vi "SlaveAccelerometerSample6.vi"   [LabVIEW 2016]
uses:
  <vilib>/rvi/Emulation/niFpgaGetClockAttributes.vi
  <vilib>/rvi/Emulation/niFpgaSctlEmulationGetInTimedLoop.vi
  <vilib>/rvi/Emulation/niFpgaEmulationReportErrorSimple.vi
  <vilib>/rvi/eio/common/nirviEmuTemplateMethod_errors.vi
  <vilib>/rvi/Emulation/niFpgaEmulationIsFPGAContextNoSignature.vi
  <vilib>/rvi/DataTransferAndStorage/Container/Common/niFpgaContainerGetUniqueNameForEmu.vi
  <vilib>/rvi/Memory/Memory_Emulation/niFpgaMemoryEmulationCacheClearOnFirstRun.vi
  <vilib>/rvi/Memory/Memory_Emulation/nirvimemoryEmulationManagerCache_MakeExclusive.vi
  <vilib>/rvi/Memory/Memory_Emulation/niFpgaMemoryEmulationValidateCache.vi
  <vilib>/rvi/Memory/Memory_Emulation/nirvimemoryEmulationManagerCache_InsertValue.vi
  <vilib>/Utility/error.llb/Clear Errors.vi
  <vilib>/rvi/Memory/Memory_Emulation/nirvimemoryEmulationManagerCache_ReleaseExclusive.vi
  <vilib>/rvi/Memory/Memory_Emulation/nirvimemoryEmulationManagerCache_GetValue.vi
  <vilib>/rvi/Memory/Memory_Emulation/nirvimemoryEmulationManagerCache_SetValue.vi
  <vilib>/rvi/Emulation/niFpgaProcessEmulError.vi
  <vilib>/rvi/errors/niFpgaSetErrorForExecOnDevCompSimple.vi
  <vilib>/rvi/eio/common/nirviEmuReportErrorAndStop.vi
  <vilib>/rvi/FIFO/Fifo_Resource/nirvififoEmulationSetSize.vi
  <vilib>/rvi/FIFO/Fifo_Resource/nirviFifoEmulationQueueMgr.vi
  <instcachedir>/0/nirviFifoEmulationQueueMgr_E5CAEC123FF24DC58D834DCA3CDAA9B5.lvgen/nirviFifoEmulationQueueMgr_E5CAEC123FF24DC58D834DCA3CDAA9B5_007.vi
  <vilib>/rvi/FIFO/Fifo_Resource/nirvififoEmulationDetermineInputValidOut.vi
  <vilib>/rvi/FIFO/Fifo_Resource/nirvififoEmulationCreateLock.vi
  <vilib>/rvi/FIFO/Fifo_Resource/nirvififoEmulationObtainLock.vi
  <vilib>/rvi/FIFO/Fifo_Resource/nirvififoEmulationReleaseLock.vi
  <vilib>/rvi/occurrence/nirviWaitOnOccurrenceBase.vi
  <vilib>/rvi/errors/nirviReportUnexpectedCaseInternalError.vi
  <vilib>/rvi/errors/nirviReportUnexpectedCaseInternalError (U32).vi
  <instcachedir>/0/nirviFifoEmulationQueueMgr_E5CAEC123FF24DC58D834DCA3CDAA9B5.lvgen/nirviFifoEmulationQueueMgr_E5CAEC123FF24DC58D834DCA3CDAA9B5_005.vi
  <vilib>/rvi/Emulation/niFpgaCriticalErrorInLSC.vi
  <vilib>/eio/EIOMethodNode/EIOMethodNode.xnode
  <vilib>/eio/EIONode/EIONode.xnode
  <vilib>/rvi/DataTransferAndStorage/Container/XNode/niFpgaContainer.xnode
  <vilib>/rvi/DataTransferAndStorage/Register/Emulation/niFpgaRegisterEmulation.vi
  <vilib>/rvi/FIFO/Fifo_Resource/nirvififoEmulationWrite.vi
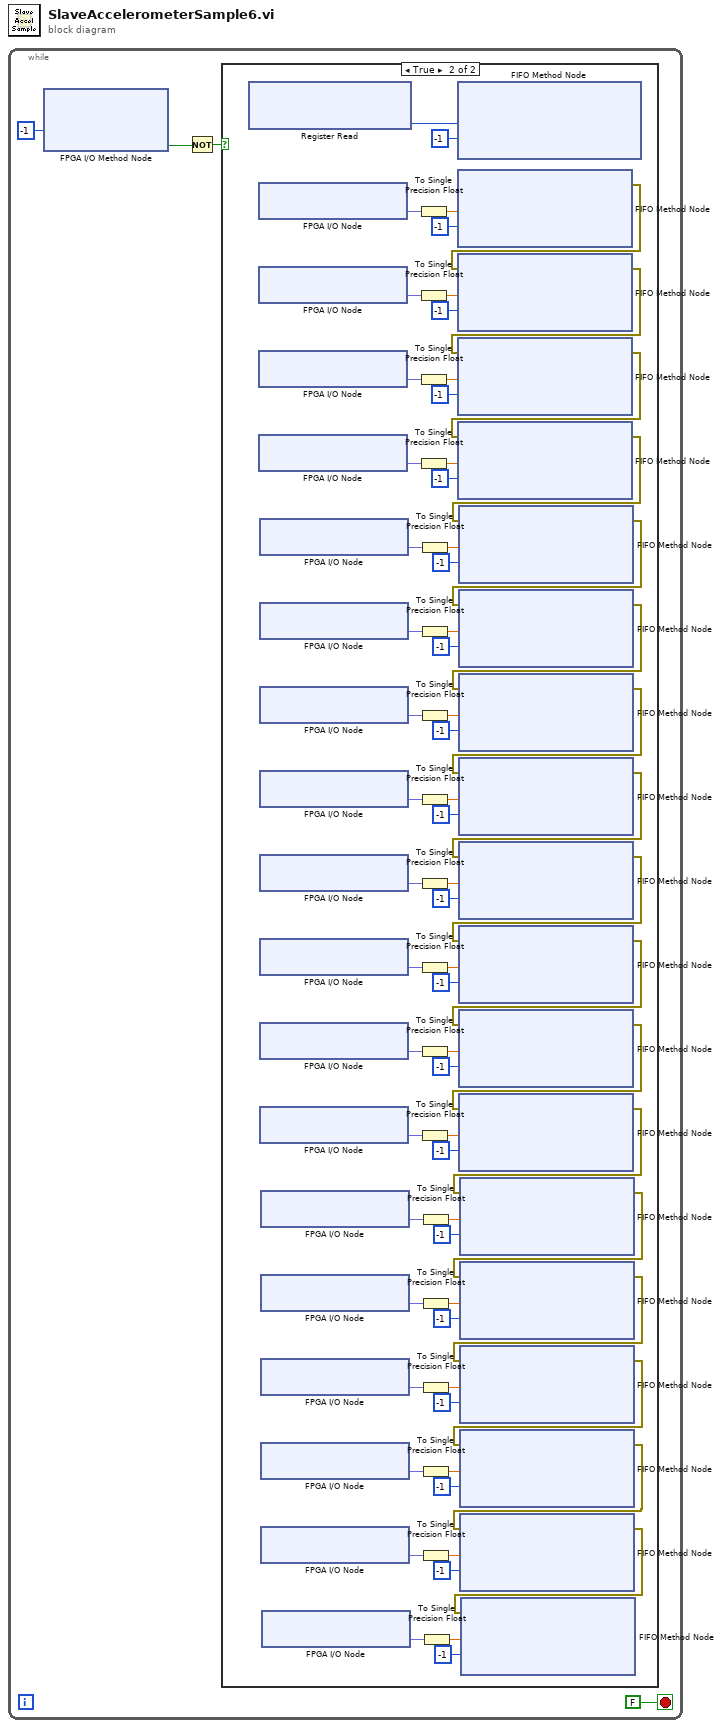
[diagram p0: block diagram]
diagram:
  n1 = while {
    stop <- FALSE stop-if-true
    n2 = xnode "FPGA I/O Method Node"("Timeout"=-1) -> ("Timed Out"=w2:bool)  [unwired: 1 in, 1 out]
    n3 = Not(x=w2) -> (.not. x?=w1:bool)
    n4 = case shown="True" w1 {
      frame False {
      }
      frame True {
        n5 = xnode "Register Read"() -> ("Data"=w5:u64)  [unwired: 1 in, 1 out]
        n6 = xnode "FPGA I/O Node"() -> ("Accelerometer1/AI0"=w76:fxp<+/-,24,7>)  [unwired: 1 in, 1 out]
        n7 = xnode "FPGA I/O Node"() -> ("Accelerometer1/AI1"=w71:fxp<+/-,24,7>)  [unwired: 1 in, 1 out]
        n8 = xnode "FPGA I/O Node"() -> ("Accelerometer1/AI2"=w63:fxp<+/-,24,7>)  [unwired: 1 in, 1 out]
        n9 = xnode "FPGA I/O Node"() -> ("Accelerometer2/AI0"=w68:fxp<+/-,24,7>)  [unwired: 1 in, 1 out]
        n10 = xnode "FPGA I/O Node"() -> ("Accelerometer2/AI1"=w47:fxp<+/-,24,7>)  [unwired: 1 in, 1 out]
        n11 = xnode "FPGA I/O Node"() -> ("Accelerometer2/AI2"=w52:fxp<+/-,24,7>)  [unwired: 1 in, 1 out]
        n12 = xnode "FPGA I/O Node"() -> ("Accelerometer3/AI0"=w60:fxp<+/-,24,7>)  [unwired: 1 in, 1 out]
        n13 = xnode "FPGA I/O Node"() -> ("Accelerometer3/AI1"=w55:fxp<+/-,24,7>)  [unwired: 1 in, 1 out]
        n14 = xnode "FPGA I/O Node"() -> ("Accelerometer3/AI2"=w15:fxp<+/-,24,7>)  [unwired: 1 in, 1 out]
        n15 = xnode "FPGA I/O Node"() -> ("Accelerometer4/AI0"=w20:fxp<+/-,24,7>)  [unwired: 1 in, 1 out]
        n16 = xnode "FPGA I/O Node"() -> ("Accelerometer4/AI1"=w28:fxp<+/-,24,7>)  [unwired: 1 in, 1 out]
        n17 = xnode "FPGA I/O Node"() -> ("Accelerometer4/AI2"=w23:fxp<+/-,24,7>)  [unwired: 1 in, 1 out]
        n18 = xnode "FPGA I/O Node"() -> ("Accelerometer5/AI0"=w44:fxp<+/-,24,7>)  [unwired: 1 in, 1 out]
        n19 = xnode "FPGA I/O Node"() -> ("Accelerometer5/AI1"=w39:fxp<+/-,24,7>)  [unwired: 1 in, 1 out]
        n20 = xnode "FPGA I/O Node"() -> ("Accelerometer5/AI2"=w31:fxp<+/-,24,7>)  [unwired: 1 in, 1 out]
        n21 = xnode "FPGA I/O Node"() -> ("Accelerometer6/AI0"=w36:fxp<+/-,24,7>)  [unwired: 1 in, 1 out]
        n22 = xnode "FPGA I/O Node"() -> ("Accelerometer6/AI1"=w13:fxp<+/-,24,7>)  [unwired: 1 in, 1 out]
        n23 = xnode "FPGA I/O Node"() -> ("Accelerometer6/AI2"=w8:fxp<+/-,24,7>)  [unwired: 1 in, 1 out]
        n24 = To Single Precision Float(number=w76) -> (single precision float=w75:sgl)
        n25 = To Single Precision Float(number=w71) -> (single precision float=w72:sgl)
        n26 = To Single Precision Float(number=w63) -> (single precision float=w64:sgl)
        n27 = To Single Precision Float(number=w68) -> (single precision float=w67:sgl)
        n28 = To Single Precision Float(number=w47) -> (single precision float=w48:sgl)
        n29 = To Single Precision Float(number=w52) -> (single precision float=w51:sgl)
        n30 = To Single Precision Float(number=w60) -> (single precision float=w59:sgl)
        n31 = To Single Precision Float(number=w55) -> (single precision float=w56:sgl)
        n32 = To Single Precision Float(number=w15) -> (single precision float=w16:sgl)
        n33 = To Single Precision Float(number=w20) -> (single precision float=w19:sgl)
        n34 = To Single Precision Float(number=w28) -> (single precision float=w27:sgl)
        n35 = To Single Precision Float(number=w23) -> (single precision float=w24:sgl)
        n36 = To Single Precision Float(number=w44) -> (single precision float=w43:sgl)
        n37 = To Single Precision Float(number=w39) -> (single precision float=w40:sgl)
        n38 = To Single Precision Float(number=w31) -> (single precision float=w32:sgl)
        n39 = To Single Precision Float(number=w36) -> (single precision float=w35:sgl)
        n40 = To Single Precision Float(number=w13) -> (single precision float=w12:sgl)
        n41 = To Single Precision Float(number=w8) -> (single precision float=w9:sgl)
        n42 = xnode ("FIFO Method Node")("Element"=w5, "Timeout"=-1) -> ()  [unwired: 1 in, 2 out]
        n43 = xnode ("FIFO Method Node")("Element"=w75, "Timeout"=-1) -> ("error out"=w70:errorcluster)  [unwired: 2 in, 2 out]
        n44 = xnode ("FIFO Method Node")("Element"=w72, "Timeout"=-1, "error in (no error)"=w70) -> ("error out"=w62:errorcluster)  [unwired: 1 in, 2 out]
        n45 = xnode ("FIFO Method Node")("Element"=w64, "Timeout"=-1, "error in (no error)"=w62) -> ("error out"=w69:errorcluster)  [unwired: 1 in, 2 out]
        n46 = xnode ("FIFO Method Node")("Element"=w67, "Timeout"=-1, "error in (no error)"=w69) -> ("error out"=w46:errorcluster)  [unwired: 1 in, 2 out]
        n47 = xnode ("FIFO Method Node")("Element"=w48, "Timeout"=-1, "error in (no error)"=w46) -> ("error out"=w53:errorcluster)  [unwired: 1 in, 2 out]
        n48 = xnode ("FIFO Method Node")("Element"=w51, "Timeout"=-1, "error in (no error)"=w53) -> ("error out"=w61:errorcluster)  [unwired: 1 in, 2 out]
        n49 = xnode ("FIFO Method Node")("Element"=w59, "Timeout"=-1, "error in (no error)"=w61) -> ("error out"=w54:errorcluster)  [unwired: 1 in, 2 out]
        n50 = xnode ("FIFO Method Node")("Element"=w56, "Timeout"=-1, "error in (no error)"=w54) -> ("error out"=w14:errorcluster)  [unwired: 1 in, 2 out]
        n51 = xnode ("FIFO Method Node")("Element"=w16, "Timeout"=-1, "error in (no error)"=w14) -> ("error out"=w21:errorcluster)  [unwired: 1 in, 2 out]
        n52 = xnode ("FIFO Method Node")("Element"=w19, "Timeout"=-1, "error in (no error)"=w21) -> ("error out"=w29:errorcluster)  [unwired: 1 in, 2 out]
        n53 = xnode ("FIFO Method Node")("Element"=w27, "Timeout"=-1, "error in (no error)"=w29) -> ("error out"=w22:errorcluster)  [unwired: 1 in, 2 out]
        n54 = xnode ("FIFO Method Node")("Element"=w24, "Timeout"=-1, "error in (no error)"=w22) -> ("error out"=w45:errorcluster)  [unwired: 1 in, 2 out]
        n55 = xnode ("FIFO Method Node")("Element"=w43, "Timeout"=-1, "error in (no error)"=w45) -> ("error out"=w38:errorcluster)  [unwired: 1 in, 2 out]
        n56 = xnode ("FIFO Method Node")("Element"=w40, "Timeout"=-1, "error in (no error)"=w38) -> ("error out"=w30:errorcluster)  [unwired: 1 in, 2 out]
        n57 = xnode ("FIFO Method Node")("Element"=w32, "Timeout"=-1, "error in (no error)"=w30) -> ("error out"=w37:errorcluster)  [unwired: 1 in, 2 out]
        n58 = xnode ("FIFO Method Node")("Element"=w35, "Timeout"=-1, "error in (no error)"=w37) -> ("error out"=w6:errorcluster)  [unwired: 1 in, 2 out]
        n59 = xnode ("FIFO Method Node")("Element"=w12, "Timeout"=-1, "error in (no error)"=w6) -> ("error out"=w7:errorcluster)  [unwired: 1 in, 2 out]
        n60 = xnode ("FIFO Method Node")("Element"=w9, "Timeout"=-1, "error in (no error)"=w7) -> ()  [unwired: 1 in, 3 out]
      }
    }
  }
